vi "MainInterface.vi"() -> ()   [LabVIEW 2015]
uses:
  <vilib>/vision/NI_Vision_Development_Module.lvlib
panel:
  out "Synchronous Display":bool
  out "x != y?":bool
  in  "appended path 2":path
  out "Image Type":T1 items=["Grayscale (U8)", "Grayscale (I16)", "Grayscale (SGL)", "Complex (CSG)", "RGB (U32)", "HSL (U32)", "RGB (U64)", "Grayscale (U16)"]
  out "run time (ms)":u32
  out "SampleStartTime":dbl
  out "Index":i32
  out "acquire period (ms)":dbl
  in  "save image":bool
  in  "sofware triffer":bool
  in  "Trigger ON":bool
  in  "live":bool
  in  "gain":i32(slide) scale=32.0..2047.0
  in  "exposure (us)":i32(slide) caption="exposure" scale=50.0..30000000.0
  out "error out":errorcluster
  in  "Stop Button":bool
  in  "?":T2(tab)
  in  "Close Device":bool
  in  "Open Device":bool
  in  "Devices found":i32(listbox)
  in  "ICImagingControl":refnum<k7>(container)
  in  "Video Format":i32(listbox)
  in  "Input Channel":i32(listbox)
  in  "Video Norm":i32(listbox)
  in  "Framerate":i32(listbox)
  in  "VCD Properties":bool
  out "Histogram":T3(graph)
  out "float image":T4(plugin-control)
  out "aquisition":T4(plugin-control)
  out "Histogram 2":T3(graph)
  out "filtered data 2":sgl[][](graph)
  out "Waveform Chart":dbl(graph)
  out "FFT":dbl[][](graph)
  out "sum On ROI":dbl
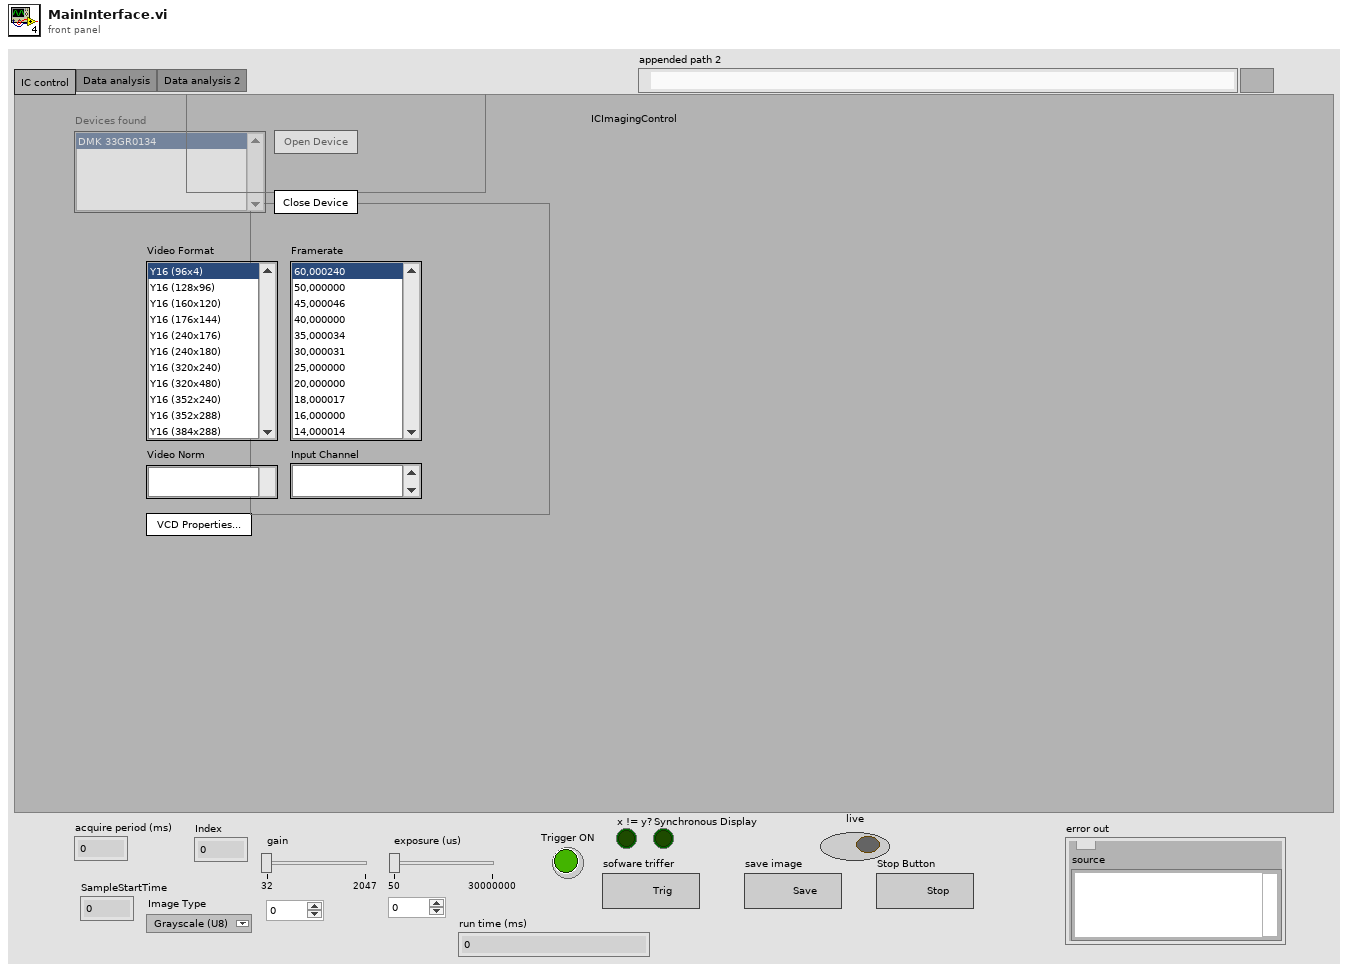
[diagram p1: front panel]
types:
  T1 = typedef "Image Type" = u32
  T2 = enum32{"IC control", "Data analysis", "Data analysis 2"}
  T3 = cluster{"Starting Value":sgl, "Incremental Value":sgl, "Histogram":u32[]}
  T4 = typedef "IMAQ Image.ctl" = refnum<image>
  T5 = enum16{"Brightness", "Color Enable", "Contrast", "Exposure", "Focus", "Gain", "Gamma", "Hue", "Iris", "Pan", "Roll", "Saturation", "Sharpness", "Tilt", "Whitebalance", "Zoom", "Whitebalance Blue", "Whitebalance Red"}
  T6 = cluster{"Rows Per Strip":i32, "Photometric":i32, "Compression Type":i32}
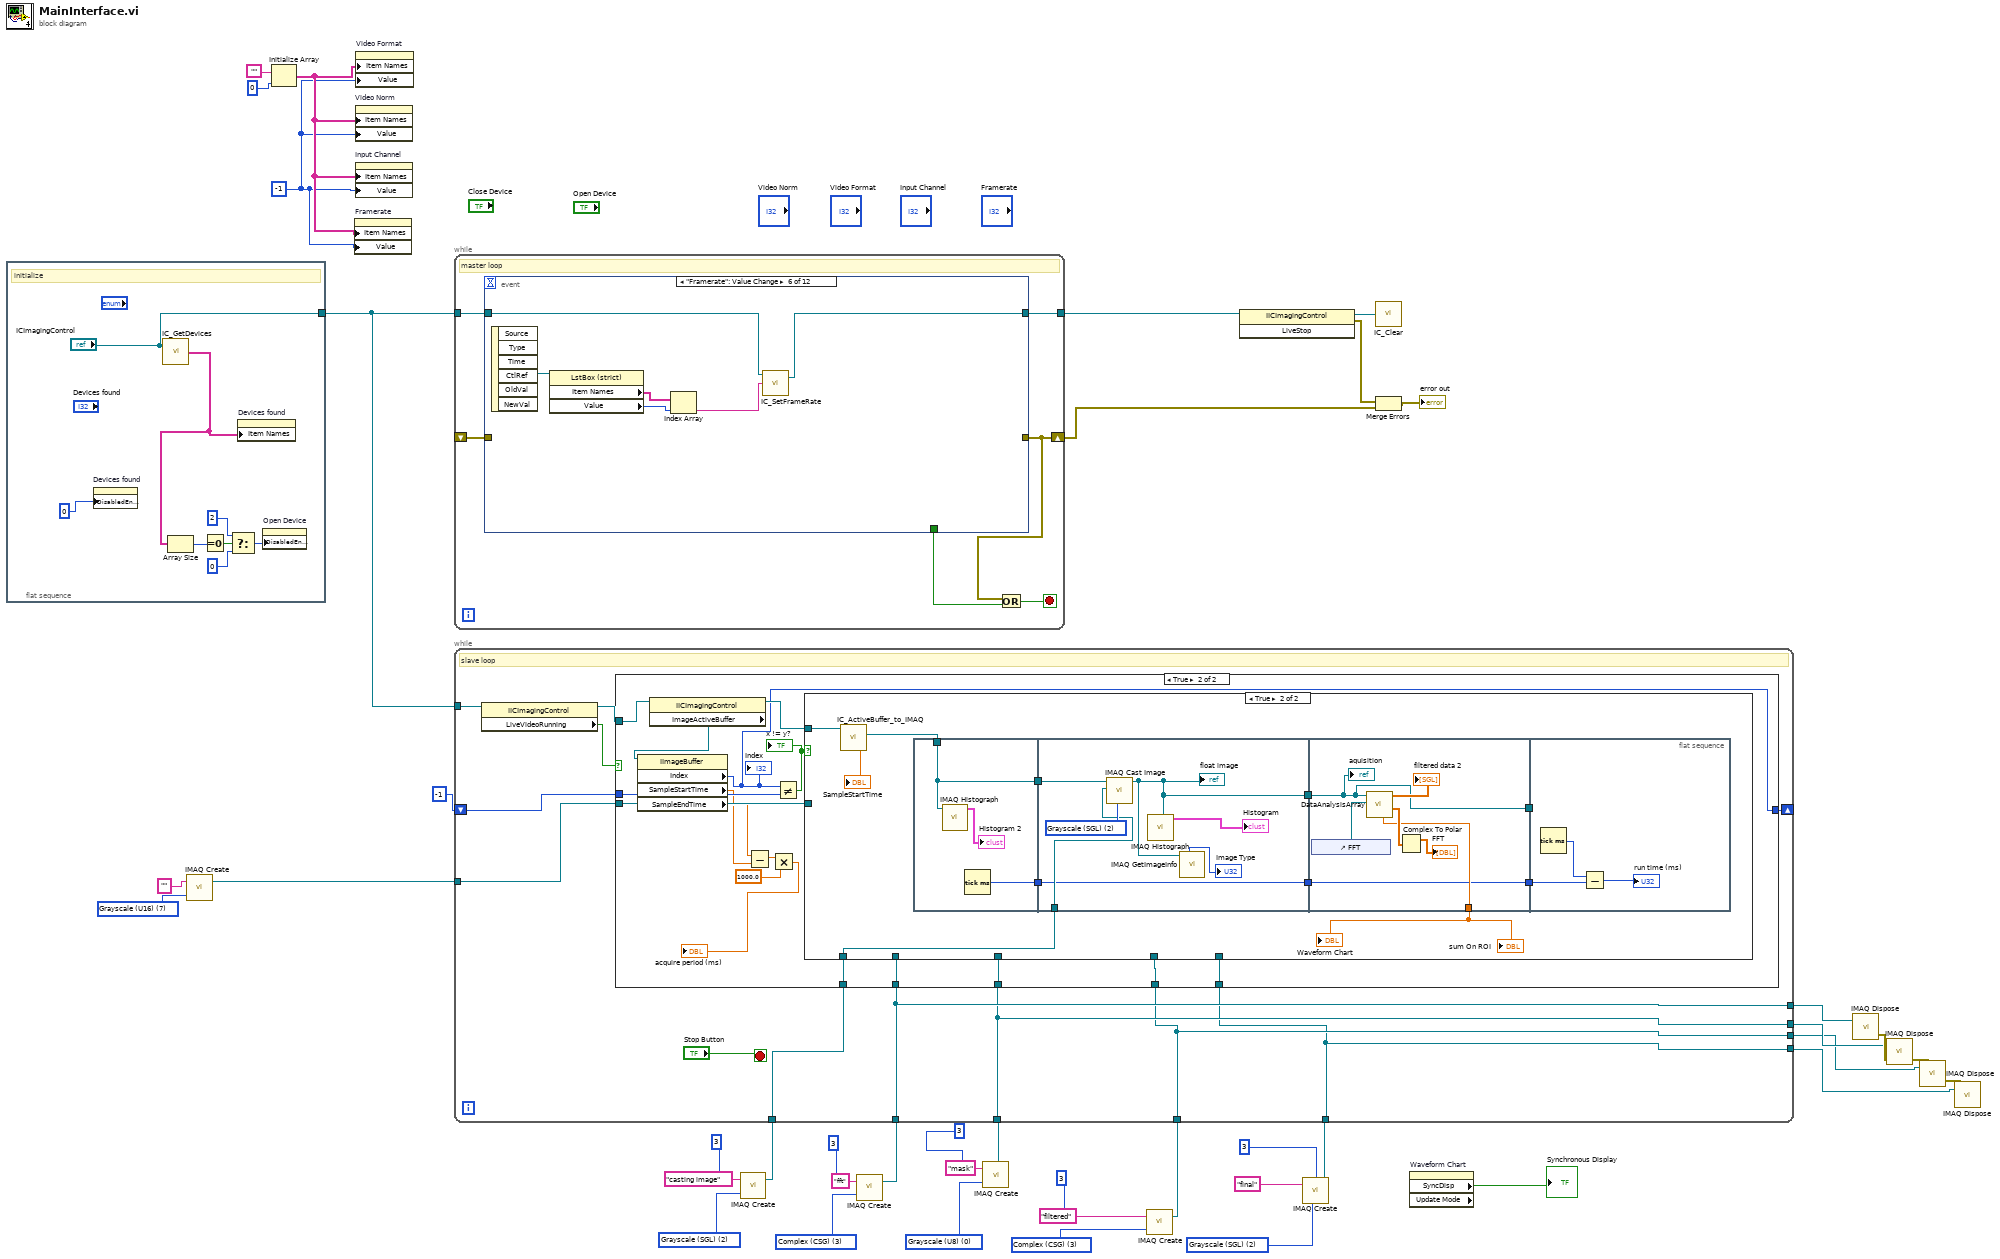
[diagram p0: block diagram]
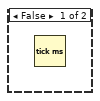
[diagram p3: hidden frame]
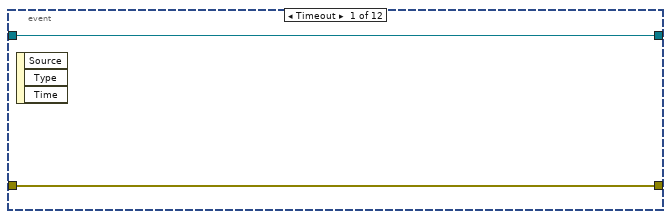
[diagram p4: hidden frame]
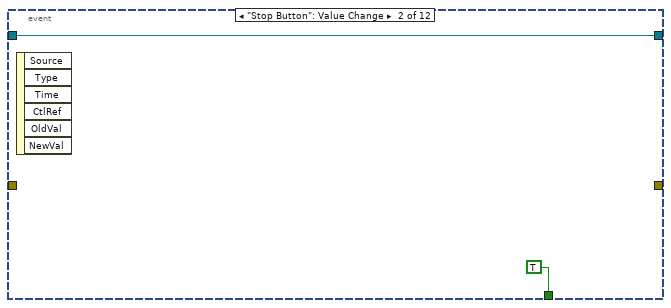
[diagram p5: hidden frame]
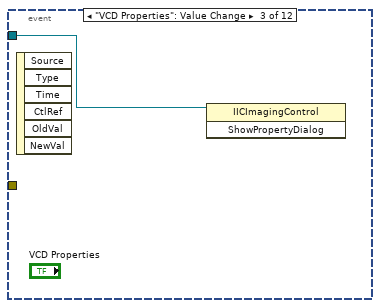
[diagram p6: hidden frame]
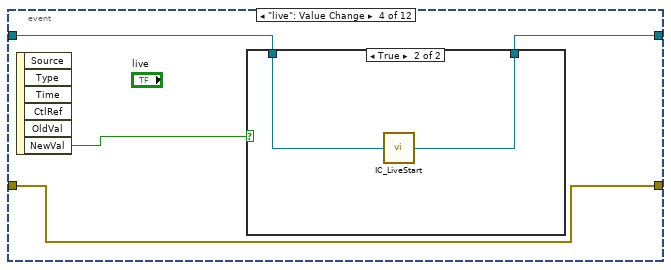
[diagram p7: hidden frame]
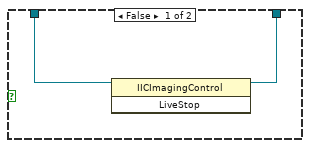
[diagram p8: hidden frame]
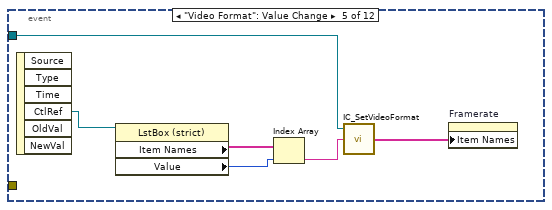
[diagram p9: hidden frame]
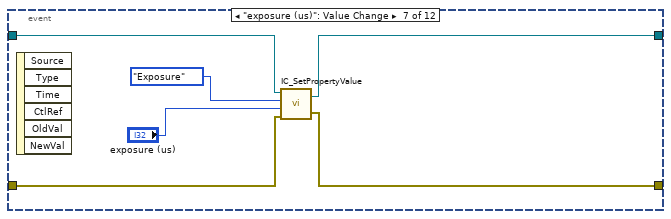
[diagram p10: hidden frame]
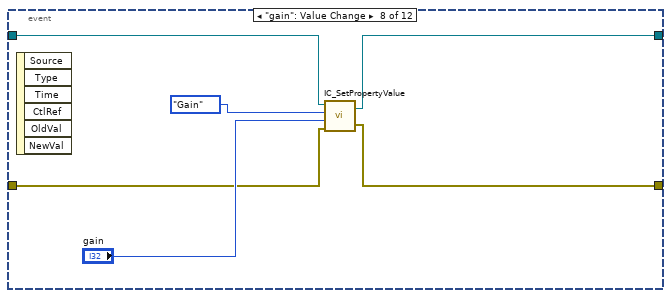
[diagram p11: hidden frame]
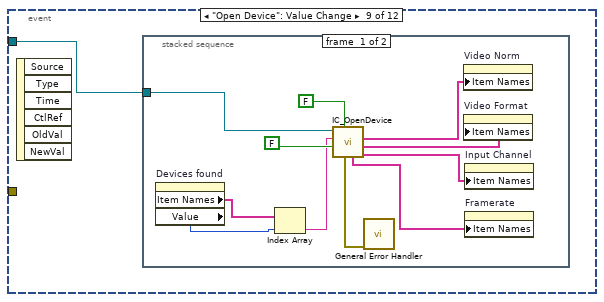
[diagram p12: hidden frame]
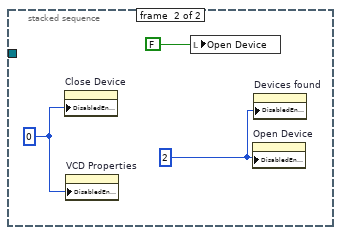
[diagram p13: hidden frame]
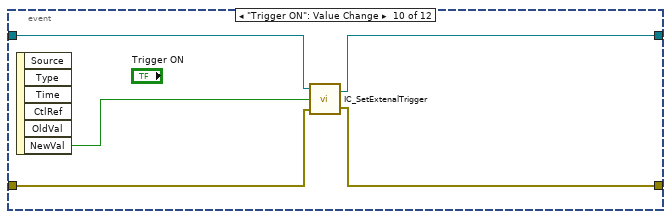
[diagram p14: hidden frame]
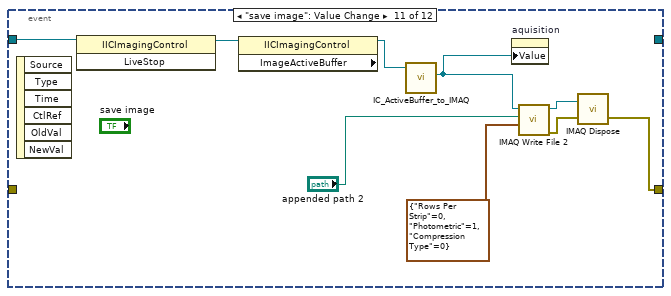
[diagram p15: hidden frame]
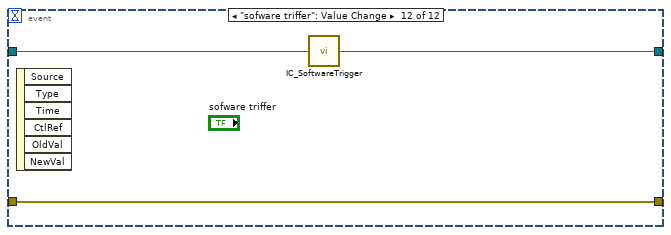
[diagram p16: hidden frame]
diagram:
  w5 = T1 2 items=["Grayscale (U8)", "Grayscale (I16)", "Grayscale (SGL)", "Complex (CSG)", "RGB (U32)", "HSL (U32)", "RGB (U64)", "Grayscale (U16)"] ("Image Type")
  w13 = -1
  w24 = T1 3 items=["Grayscale (U8)", "Grayscale (I16)", "Grayscale (SGL)", "Complex (CSG)", "RGB (U32)", "HSL (U32)", "RGB (U64)", "Grayscale (U16)"] ("Image Type")
  w28 = T1 2 items=["Grayscale (U8)", "Grayscale (I16)", "Grayscale (SGL)", "Complex (CSG)", "RGB (U32)", "HSL (U32)", "RGB (U64)", "Grayscale (U16)"] ("Image Type")
  w32 = T1 0 items=["Grayscale (U8)", "Grayscale (I16)", "Grayscale (SGL)", "Complex (CSG)", "RGB (U32)", "HSL (U32)", "RGB (U64)", "Grayscale (U16)"] ("Image Type")
  w34 = T1 7 items=["Grayscale (U8)", "Grayscale (I16)", "Grayscale (SGL)", "Complex (CSG)", "RGB (U32)", "HSL (U32)", "RGB (U64)", "Grayscale (U16)"] ("Image Type")
  w39 = T1 3 items=["Grayscale (U8)", "Grayscale (I16)", "Grayscale (SGL)", "Complex (CSG)", "RGB (U32)", "HSL (U32)", "RGB (U64)", "Grayscale (U16)"] ("Image Type")
  n1 = flat-sequence {
    tunnel: ["ICImagingControl"] -> w17
    frame #0 {
      # "initialize"
      n2 = property on="Devices found" class="LstBox (strict)"("DisabledEnum"=u8 0 ("Disabled")) -> ()  [unwired: 2 in, 2 out]
      n3 = call <userlib>:"IC_GetDevices.vi"("ICImagingControl In"="ICImagingControl") -> ("Devices"=w46:string[])  [unwired: 1 in, 2 out]
      n4 = Array Size(array=w46) -> (size(s)=w50:i32)
      n5 = Equal To 0?(x=w50) -> (x = 0?=w49:bool)
      n6 = Select(t=u8 2 ("Disabled"), s=w49, f=u8 0 ("Disabled")) -> (s? t:f=w45:u8)
      n7 = property on="Devices found" class="LstBox (strict)"("Item Names"=w46) -> ()  [unwired: 2 in, 2 out]
      n8 = property on="Open Device" class="Bool (strict)"("DisabledEnum"=w45) -> ()  [unwired: 2 in, 2 out]
    }
  }
  n9 = call "IMAQ Create"("Image Name"="", "Image Type"=w34) -> ("New Image"=w33:T4)  [unwired: 3 in, 1 out]
  n10 = Initialize Array("", 0) -> (w14:string[])
  n11 = property on="Framerate" class="LstBox (strict)"("Item Names"=w14, "Value"=w13) -> ()  [unwired: 2 in, 2 out]
  n12 = property on="Video Norm" class="LstBox (strict)"("Item Names"=w14, "Value"=w13) -> ()  [unwired: 2 in, 2 out]
  n13 = property on="Input Channel" class="LstBox (strict)"("Item Names"=w14, "Value"=w13) -> ()  [unwired: 2 in, 2 out]
  n14 = property on="Video Format" class="LstBox (strict)"("Item Names"=w14, "Value"=w13) -> ()  [unwired: 2 in, 2 out]
  n15 = while {
    tunnel: w17 -> [w55]
    tunnel: [w56] -> w42
    shift-right: [w53] -> w20
    shift-left: _ -> [w54]
    stop <- w52 stop-if-true
    # "master loop"
    n16 = event shown="[5] \"Framerate\": Value Change" {
      selector: _ -> [_ _ _ _ _ _ _ _ _ _ _ _]
      dyn-events: _ -> [_ _ _ _ _ _ _ _ _ _ _ _]
      timeout: _ -> [_ _ _ _ _ _ _ _ _ _ _ _]
      tunnel: [_ TRUE _ _ _ _ _ _ _ _ _ _] -> w51
      tunnel: [w57 w59 _ w62 _ w76 w86 w89 _ w112 _ w124] -> w56
      tunnel: w55 -> [w57 w59 w61 w63 w75 w80 w87 w88 w94 w113 w117 w125]
      tunnel: [w58 _ _ w64 _ _ w84 w90 _ w111 w121 w123] -> w53
      tunnel: w54 -> [w58 _ _ w64 _ _ w85 w91 _ w110 _ w123]
      event Timeout {
        n17 = event-data() -> ()  [unwired: 1 in, 3 out]
      }
      event "Stop Button": Value Change {
        n18 = event-data() -> ()  [unwired: 1 in, 6 out]
      }
      event "VCD Properties": Value Change {
        n19 = event-data() -> ()  [unwired: 1 in, 6 out]
        n20 = invoke class="IICImagingControl" method="ShowPropertyDialog"(reference=w61) -> ()  [unwired: 2 in, 3 out]
      }
      event "live": Value Change {
        n21 = event-data() -> ("NewVal"=w65:bool)  [unwired: 1 in, 5 out]
        n22 = case shown="True" w65 {
          tunnel: w63 -> [w67 w69]
          tunnel: [w66 w68] -> w62
          frame False {
            n23 = invoke class="IICImagingControl" method="LiveStop"(reference=w67) -> (reference out=w66:refnum<k7>)  [unwired: 2 in, 2 out]
          }
          frame True {
            n24 = call <userlib>:"IC_LiveStart.vi"("ICImagingControl 3"=w69) -> ("ICImagingControl 2"=w68:refnum<k7>)
          }
        }
      }
      event "Video Format": Value Change {
        n25 = event-data() -> ("CtlRef"=w74:refnum<vi>)  [unwired: 1 in, 5 out]
        n26 = property class="LstBox (strict)"(reference=w74) -> ("Item Names"=w73:string[], "Value"=w72:i32)  [unwired: 1 in, 2 out]
        n27 = Index Array(array=w73, index=w72) -> (element=w71:string)
        n28 = call <userlib>:"IC_SetVideoFormat.vi"("VideoFormat"=w71, "ICImagingControl In"=w75) -> ("FrameRates"=w70:string[])  [unwired: 1 in, 2 out]
        n29 = property on="Framerate" class="LstBox (strict)"("Item Names"=w70) -> ()  [unwired: 2 in, 2 out]
      }
      event "Framerate": Value Change {
        n30 = event-data() -> ("CtlRef"=w81:refnum<vi>)  [unwired: 1 in, 5 out]
        n31 = property class="LstBox (strict)"(reference=w81) -> ("Item Names"=w79:string[], "Value"=w78:i32)  [unwired: 1 in, 2 out]
        n32 = Index Array(array=w79, index=w78) -> (element=w77:string)
        n33 = call <userlib>:"IC_SetFrameRate.vi"("FrameRate"=w77, "ICImagingControl In"=w80) -> ("ICImagingControl Out"=w76:refnum<k7>)  [unwired: 1 in, 1 out]
      }
      event "exposure (us)": Value Change {
        n34 = event-data() -> ()  [unwired: 1 in, 6 out]
        n35 = call <userlib>:"IC_SetPropertyValue.vi"("Error In (no error)"=w85, "Value"="exposure (us)", "Property"=T5."Exposure", "ICImagingControl In"=w87) -> ("Error Out"=w84:errorcluster, "ICImagingControl Out"=w86:refnum<k7>)
      }
      event "gain": Value Change {
        n36 = event-data() -> ()  [unwired: 1 in, 6 out]
        n37 = call <userlib>:"IC_SetPropertyValue.vi"("Error In (no error)"=w91, "Value"="gain", "Property"=T5."Gain", "ICImagingControl In"=w88) -> ("Error Out"=w90:errorcluster, "ICImagingControl Out"=w89:refnum<k7>)
      }
      event "Open Device": Value Change {
        n38 = event-data() -> ()  [unwired: 1 in, 6 out]
        n39 = stacked-sequence {
          tunnel: w94 -> [w103 _]
          frame #0 {
            n40 = property on="Devices found" class="LstBox (strict)"() -> ("Item Names"=w105:string[], "Value"=w104:i32)  [unwired: 2 in, 2 out]
            n41 = Index Array(array=w105, index=w104) -> (element=w100:string)
            n42 = call <userlib>:"IC_OpenDevice.vi"("Color"=FALSE, "Live"=FALSE, "Device"=w100, "ICImagingControl In"=w103) -> ("InputChannels"=w97:string[], "VideoFormats"=w96:string[], "VideoNorms"=w95:string[], "FrameRates"=w98:string[], "Error Out"=w99:errorcluster)  [unwired: 2 in, 1 out]
            n43 = call <vilib>:"General Error Handler.vi"("error in (no error)"=w99) -> ()  [unwired: 10 in, 5 out]
            n44 = property on="Video Norm" class="LstBox (strict)"("Item Names"=w95) -> ()  [unwired: 2 in, 2 out]
            n45 = property on="Video Format" class="LstBox (strict)"("Item Names"=w96) -> ()  [unwired: 2 in, 2 out]
            n46 = property on="Input Channel" class="LstBox (strict)"("Item Names"=w97) -> ()  [unwired: 2 in, 2 out]
            n47 = property on="Framerate" class="LstBox (strict)"("Item Names"=w98) -> ()  [unwired: 2 in, 2 out]
          }
          frame #1 {
            w107 = 2
            w108 = 0
            n48 = property on="Close Device" class="Bool (strict)"("DisabledEnum"=w108) -> ()  [unwired: 2 in, 2 out]
            n49 = property on="VCD Properties" class="Bool"("DisabledEnum"=w108) -> ()  [unwired: 2 in, 2 out]
            n50 = local write "Open Device"(FALSE) -> ()
            n51 = property on="Open Device" class="Bool (strict)"("DisabledEnum"=w107) -> ()  [unwired: 2 in, 2 out]
            n52 = property on="Devices found" class="LstBox (strict)"("DisabledEnum"=w107) -> ()  [unwired: 2 in, 2 out]
          }
        }
      }
      event "Trigger ON": Value Change {
        n53 = event-data() -> ("NewVal"=w109:bool)  [unwired: 1 in, 5 out]
        n54 = call <userlib>:"IC_SetExtenalTrigger.vi"("Error In (no error)"=w110, "Trigger"=w109, "ICImagingControl In"=w113) -> ("Error Out"=w111:errorcluster, "ICImagingControl Out"=w112:refnum<k7>)
      }
      event "save image": Value Change {
        n55 = event-data() -> ()  [unwired: 1 in, 6 out]
        n56 = invoke class="IICImagingControl" method="LiveStop"(reference=w117) -> (reference out=w116:refnum<k7>)  [unwired: 2 in, 2 out]
        n57 = property class="IICImagingControl" props=["ImageActiveBuffer"](reference=w116) -> (reference out=w115:refnum<k7>)  [unwired: 1 in, 2 out]
        n58 = call <userlib>:"IC_ActiveBuffer_to_IMAQ.vi"("ICImagingControl In"=w115) -> ("Image Out"=w114:T4)  [unwired: 2 in, 3 out]
        n59 = property on="aquisition" class="ImageControl"("Value"=w114) -> ()  [unwired: 2 in, 2 out]
        n60 = call-poly "IMAQ Write File 2"("TIFF Options"=T6 {"Rows Per Strip"=0, "Photometric"=1, "Compression Type"=0}, "File Path"="appended path 2", "Image"=w114) -> ("error out"=w122:errorcluster, "Image Out (duplicate)"=w120:T4)  [unwired: 7 in]
        n61 = call "IMAQ Dispose"("Image"=w120, "error in (no error)"=w122) -> ("error out"=w121:errorcluster)  [unwired: 4 in]
      }
      event "sofware triffer": Value Change {
        n62 = event-data() -> ()  [unwired: 1 in, 6 out]
        n63 = call <userlib>:"IC_SoftwareTrigger.vi"("ICImagingControl 3"=w125) -> ("ICImagingControl 2"=w124:refnum<k7>)
      }
    }
    n64 = Or(x=w53, y=w51) -> (x .or. y?=w52:bool)
  }
  n65 = call "IMAQ Create"("Border Size"=3 ("BorderSize"), "Image Name"="casting image", "Image Type"=w5) -> ("New Image"=w2:T4)  [unwired: 2 in, 1 out]
  n66 = call "IMAQ Create"("Border Size"=3 ("BorderSize"), "Image Name"="fft", "Image Type"=w39) -> ("New Image"=w36:T4)  [unwired: 2 in, 1 out]
  n67 = call "IMAQ Create"("Border Size"=3 ("BorderSize"), "Image Name"="mask", "Image Type"=w32) -> ("New Image"=w29:T4)  [unwired: 2 in, 1 out]
  n68 = call "IMAQ Create"("Border Size"=3 ("BorderSize"), "Image Name"="filtered", "Image Type"=w24) -> ("New Image"=w21:T4)  [unwired: 2 in, 1 out]
  n69 = invoke class="IICImagingControl" method="LiveStop"(reference=w42) -> (reference out=w41:refnum<k7>, error out=w19:errorcluster)  [unwired: 2 in, 1 out]
  n70 = call "IMAQ Create"("Border Size"=3 ("BorderSize"), "Image Name"="final", "Image Type"=w28) -> ("New Image"=w25:T4)  [unwired: 2 in, 1 out]
  n71 = while {
    tunnel: w17 -> [w136]
    shift-right: [w126] -> _
    shift-left: -1 ("Index") -> [w137]
    tunnel: w36 -> [w131]
    tunnel: w33 -> [w133]
    tunnel: w29 -> [w130]
    tunnel: w25 -> [w128]
    tunnel: w21 -> [w129]
    tunnel: [w131] -> w12
    tunnel: [w130] -> w10
    tunnel: [w129] -> w9
    tunnel: [w128] -> w7
    tunnel: w2 -> [w127]
    stop <- "Stop Button" stop-if-true
    # "slave loop"
    n72 = property class="IICImagingControl"(reference=w136) -> (reference out=w135:refnum<k7>, "LiveVideoRunning"=w134:bool)  [unwired: 1 in, 1 out]
    n73 = case shown="True" w134 {
      tunnel: w137 -> [w138 w155]
      tunnel: w135 -> [_ w153]
      tunnel: w133 -> [_ w150]
      tunnel: w131 -> [_ w149]
      tunnel: w130 -> [_ w148]
      tunnel: w128 -> [_ w147]
      tunnel: w129 -> [_ w146]
      tunnel: w127 -> [_ w140]
      tunnel: [w138 w139] -> w126
      frame False {
      }
      frame True {
        n74 = property class="IICImagingControl"(reference=w153) -> (reference out=w151:refnum<k7>, "ImageActiveBuffer"=w152:refnum<k7>)  [unwired: 1 in, 1 out]
        n75 = property class="IImageBuffer"(reference=w152) -> ("Index"=w139:i32, "SampleStartTime"=w144:dbl, "SampleEndTime"=w145:dbl)  [unwired: 1 in, 2 out]
        "Index" <- w139
        n76 = Subtract(x=w145, y=w144) -> (x-y=w143:dbl)
        n77 = Multiply(x=w143, y=1000.0) -> (x*y=→"acquire period (ms)":dbl)
        n78 = Not Equal?(x=w139, y=w155) -> (x != y?=w154:bool)
        "x != y?" <- w154
        n79 = case shown="True" w154 {
          tunnel: w151 -> [_ w166]
          tunnel: w150 -> [_ _]
          tunnel: w149 -> [_ _]
          tunnel: w148 -> [_ _]
          tunnel: w147 -> [_ _]
          tunnel: w146 -> [_ _]
          tunnel: w140 -> [_ w163]
          frame False {
            n80 = Tick Count (ms)() -> ()  [unwired: 1 out]
          }
          frame True {
            n81 = call <userlib>:"IC_ActiveBuffer_to_IMAQ.vi"("ICImagingControl In"=w166) -> ("Image Out"=w164:T4, "SampleStartTime"=→"SampleStartTime":dbl)  [unwired: 2 in, 2 out]
            n82 = flat-sequence {
              tunnel: w164 -> [w168]
              tunnel: [w168] -> w162
              tunnel: [w167] -> w156
              tunnel: w163 -> [w173]
              tunnel: w162 -> [w172]
              tunnel: [w171] -> w161
              tunnel: [w170] -> w157
              tunnel: w156 -> [w170]
              tunnel: w161 -> [w178]
              tunnel: [w179] -> w160
              tunnel: [w178] -> w159
              tunnel: [w177] -> w158
              tunnel: w157 -> [w177]
              tunnel: w159 -> [_]
              tunnel: w158 -> [w185]
              frame #0 {
                n83 = call "IMAQ Histograph"("Image"=w168) -> ("Histogram Graph"=→"Histogram 2":T3)  [unwired: 7 in, 3 out]
                n84 = Tick Count (ms)() -> (millisecond timer value=w167:u32)
              }
              frame #1 {
                w176 = T1 2 items=["Grayscale (U8)", "Grayscale (I16)", "Grayscale (SGL)", "Complex (CSG)", "RGB (U32)", "HSL (U32)", "RGB (U64)", "Grayscale (U16)"] ("Image Type")
                n85 = call "IMAQ Cast Image"("Image Type"=w176, "Image Dst"=w173, "Image Src"=w172) -> ("Image Dst Out"=w171:T4)  [unwired: 7 in, 1 out]
                "float image" <- w171
                n86 = call "IMAQ Histograph"("Image"=w171) -> ("Histogram Graph"=→"Histogram":T3)  [unwired: 7 in, 3 out]
                n87 = call "IMAQ GetImageInfo"("Image"=w171) -> ("Image Type"=→"Image Type":T1)  [unwired: 3 in, 7 out]
              }
              frame #2 {
                n88 = control-ref of="FFT"() -> (w180:refnum<vi>)
                n89 = call "DataAnalysisArray.vi"("FFT 2"=w180, "Image IN"=w178) -> ("FFT {X}"=w182:cdb[][], "Image Pixels (Float)"=→"filtered data 2":sgl[][], "sum On ROI"=w179:dbl)  [unwired: 5 in, 2 out]
                n90 = Complex To Polar(r * e^(i*theta)=w182) -> (r=→"FFT":dbl[][])  [unwired: 1 out]
                "aquisition" <- w178
              }
              frame #3 {
                n91 = Tick Count (ms)() -> (millisecond timer value=w186:u32)
                n92 = Subtract(x=w186, y=w185) -> (x-y=→"run time (ms)":u32)
              }
            }
            "Waveform Chart" <- w160
            "sum On ROI" <- w160
          }
        }
      }
    }
  }
  n93 = call <userlib>:"IC_Clear.vi"("ICImagingControl 2"=w41) -> ()  [unwired: 1 out]
  n94 = Merge Errors(w19, w20) -> (→"error out":errorcluster)
  n95 = property on="Waveform Chart" class="WFChart (strict)" props=["SyncDisp", "Update Mode"]() -> ("SyncDisp"=→"Synchronous Display":bool)  [unwired: 2 in, 3 out]
  n96 = call "IMAQ Dispose"("Image"=w12) -> ("error out"=w11:errorcluster)  [unwired: 5 in]
  n97 = call "IMAQ Dispose"("Image"=w10, "error in (no error)"=w11) -> ("error out"=w8:errorcluster)  [unwired: 4 in]
  n98 = call "IMAQ Dispose"("Image"=w9, "error in (no error)"=w8) -> ("error out"=w6:errorcluster)  [unwired: 4 in]
  n99 = call "IMAQ Dispose"("Image"=w7, "error in (no error)"=w6) -> ()  [unwired: 4 in, 1 out]
